vi "Set Measurement Name.vi"(8 "error in (no error)":errorcluster, 11 "ModSweep in":refnum<class "ModSweep.lvclass">) -> (0 "error out":errorcluster, 3 "ModSweep out":refnum<class "ModSweep.lvclass">)   [LabVIEW 2018, in "ModSweep.lvlib" / "ModSweep.lvclass"]
uses:
  ModSweep.lvclass
  Plugins/String Database.lvlibp/String Database.lvclass
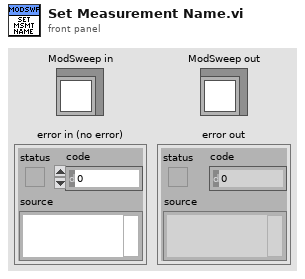
[diagram p1: front panel]
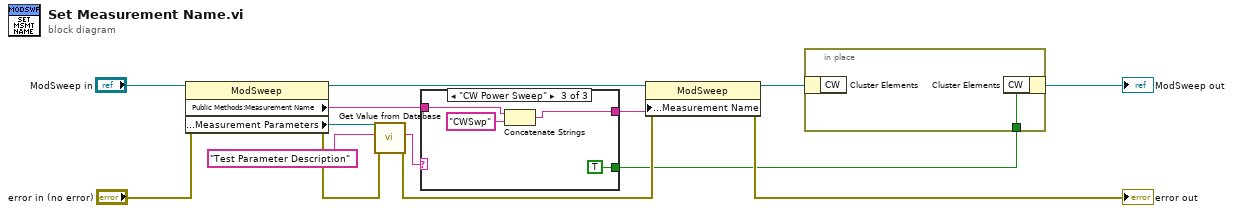
[diagram p0: block diagram]
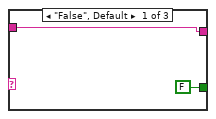
[diagram p2: hidden frame]
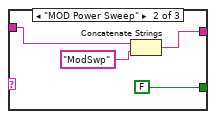
[diagram p3: hidden frame]
diagram:
  n1 = property class="ModSweep"(reference="ModSweep in", error in="error in (no error)") -> (reference out=w11:refnum<class "ModSweep.lvclass">, error out=w8:errorcluster, "Public Methods:Measurement Name"=w13:string, "Protected Methods:Measurement Parameters"=w9:refnum<class "String Database.lvclass">)
  n2 = call "Get Value from Database.vi"("error in (no error)"=w8, "Entry Name"="Test Parameter Description", "Message in"=w9) -> ("error out"=w7:errorcluster, "Entry Value"=w5:string)  [unwired: 5 in, 2 out]
  n3 = case shown="\"CW Power Sweep\"" w5 {
    tunnel: w13 -> [w16 w20 w23]
    tunnel: [w16 w18 w24] -> w10
    tunnel: [FALSE FALSE TRUE] -> w2
    frame "False", Default {
    }
    frame "MOD Power Sweep" {
      n4 = Concatenate Strings(w20, "ModSwp" ("string")) -> (w18:string)
    }
    frame "CW Power Sweep" {
      n5 = Concatenate Strings(w23, "CWSwp" ("string")) -> (w24:string)
    }
  }
  n6 = property class="ModSweep"(reference=w11, error in=w7, "Public Methods:Measurement Name"=w10) -> (reference out=w4:refnum<class "ModSweep.lvclass">, error out=→"error out":errorcluster)
  n7 = in-place {
    in-place-border: w2 -> [w25]
    n8 = in-place-cluster #1(w4) -> ()  [unwired: 1 out]
    n9 = in-place-cluster #1("CW"=w25) -> (→"ModSweep out":refnum<class "ModSweep.lvclass">)
  }
